vi "Tab Controls.vi"() -> ()   [LabVIEW 2024]
panel:
  in  "Tab Control":T1(tab)
  in  "Numeric 4":dbl
  in  "Numeric 3":dbl
  in  "Numeric 2":dbl
  in  "Numeric":dbl
  out "Waveform Chart":dbl(graph)
  out "Intensity Graph":dbl[][](graph)
  out "Digital Waveform Graph":T2(graph)
  # "Overview: Usage of Tab Controls and used Decorations\n\nTab controls are used to switch between the pages similar to web pages\nRight click ->Numeric->Layout - >Tab control\nRight click ->Numeric->Decorations"
  # "."
  # "OUTPUT"
  # "INPUT"
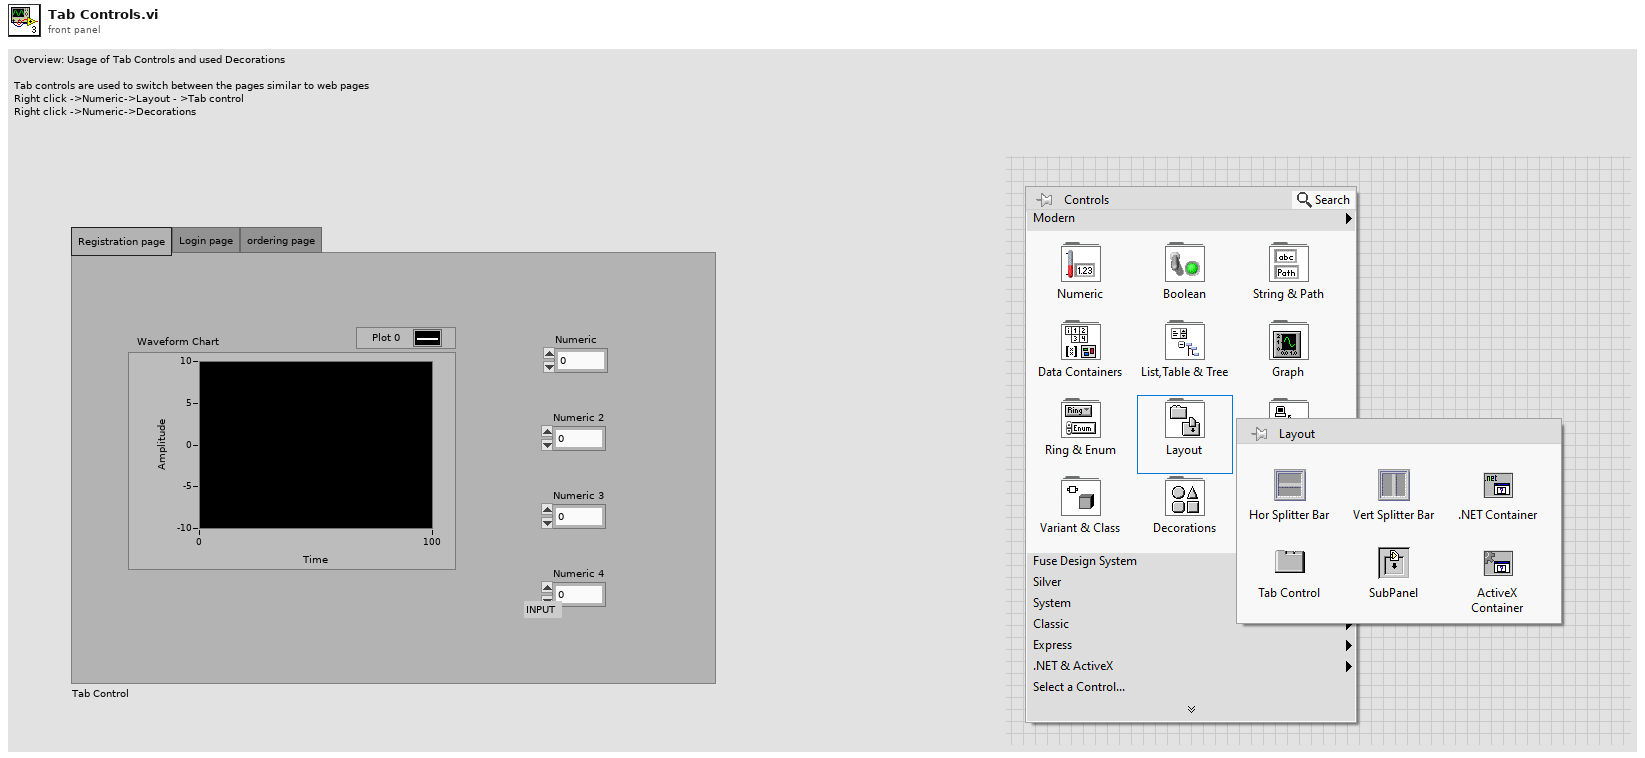
[diagram p1: front panel]
types:
  T1 = enum32{"Registration page", "Login page", "ordering page"}
  T2 = cluster{"x0":dbl, "dx":dbl, "[y]":u8[], "ports":i32}
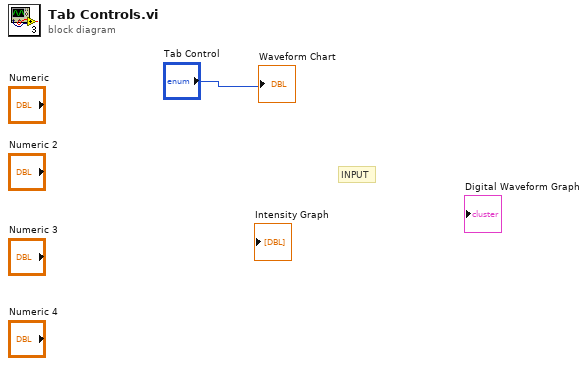
[diagram p0: block diagram]
diagram:
  # "INPUT"
  "Waveform Chart" <- "Tab Control"
